vi "DriveModuleControl.vi"(8 "error in":errorcluster, 9 "Actual State":T1={"Speed"=0.0, "Angle"={"VALUE"=0.0, "COS"=1.0, "SIN"=0.0}} {"Angle"."SIN" format="%13.4f"; "Angle"."COS" format="%13.4f"; "Angle"."VALUE" format="%13.4f"}, 10 "Desired State":T1={"Speed"=0.0, "Angle"={"VALUE"=0.0, "COS"=1.0, "SIN"=0.0}} {"Angle"."SIN" format="%13.4f"; "Angle"."COS" format="%13.4f"; "Angle"."VALUE" format="%13.4f"}, 11 "ModualNamePrefix":i32) -> (0 "error out":errorcluster)   [LabVIEW 2023]
uses:
  <vilib>/Rock Robotics/WPI/ThirdParty/JAS_Junk/TrajLib/TypeDef/SWERVE_DRIVE_MODULE_STATE.ctl
  <vilib>/Rock Robotics/WPI/ThirdParty/JAS_Junk/TrajLib/TypeDef/ROTATION2D.ctl
  <vilib>/Rock Robotics/WPI/ThirdParty/JAS_Junk/TrajLib/Rotation2d_Minus.vi
  <vilib>/Rock Robotics/WPI/ThirdParty/JAS_Junk/TrajLib/Rotation2d_GetRadians.vi
  <vilib>/Rock Robotics/WPI/ThirdParty/JAS_Junk/TrajLib/SwerveModuleState_New.vi
  <vilib>/Rock Robotics/WPI/ThirdParty/JAS_Junk/TrajLib/Rotation2d_RotateBy.vi
  <vilib>/Rock Robotics/WPI/ThirdParty/JAS_Junk/TrajLib/Rotation2d_CreateAngle.vi
  <vilib>/Rock Robotics/WPI/ThirdParty/JAS_Junk/TrajLib/SimpleMotorFF_Calculate.vi
  <vilib>/Rock Robotics/WPI/ThirdParty/JAS_Junk/TrajLib/PIDController_AtSetpoint.vi
  <vilib>/Rock Robotics/WPI/ThirdParty/JAS_Junk/TrajLib/PIDController_SetPIDF.vi
  <vilib>/Rock Robotics/WPI/ThirdParty/JAS_Junk/TrajLib/PIDController_SetDerivativeFilter.vi
  <vilib>/Rock Robotics/WPI/ThirdParty/JAS_Junk/TrajLib/PIDController_SetIntegratorRange.vi
  <vilib>/Rock Robotics/WPI/ThirdParty/JAS_Junk/TrajLib/PIDController_SetTolerancePandV.vi
  <vilib>/Rock Robotics/WPI/ThirdParty/JAS_Junk/TrajLib/PIDController_DisableContinousInput.vi
  <vilib>/Rock Robotics/WPI/ThirdParty/JAS_Junk/TrajLib/PIDController_EnableContinousInput.vi
  <vilib>/Rock Robotics/WPI/ThirdParty/JAS_Junk/TrajLib/PIDController_Reset.vi
  <vilib>/Rock Robotics/WPI/ThirdParty/JAS_Junk/TrajLib/PIDController_New.vi
  <vilib>/Rock Robotics/WPI/ThirdParty/JAS_Junk/TrajLib/PIDController_SetOutputLimits.vi
  <vilib>/Rock Robotics/WPI/ThirdParty/JAS_Junk/TrajLib/VI/PIDController_SetIntegratorZone.vi
  <vilib>/Rock Robotics/WPI/ThirdParty/JAS_Junk/TrajLib/SlewRateLimiter_New.vi
  <vilib>/Rock Robotics/WPI/ThirdParty/JAS_Junk/TrajLib/SlewRateLimiter_Reset.vi
  <vilib>/Rock Robotics/WPI/ThirdParty/JAS_Junk/TrajLib/SlewRateLimiter_Calculate.vi
  <vilib>/Rock Robotics/WPI/ThirdParty/JAS_Junk/TrajLib/SlewRateLimiter_SetRate.vi
  <vilib>/Rock Robotics/WPI/ThirdParty/JAS_Junk/TrajLib/Rotation2d_UnaryMinus.vi
  <vilib>/Rock Robotics/WPI/ThirdParty/JAS_Junk/TrajLib/Rotation2d_CreateXY.vi
  <vilib>/Rock Robotics/WPI/ThirdParty/JAS_Junk/TrajLib/PIDController_NewPeriod.vi
  <vilib>/Rock Robotics/WPI/ThirdParty/JAS_Junk/TrajLib/Util_GetTime.vi
  <vilib>/Rock Robotics/WPI/ThirdParty/JAS_Junk/TrajLib/Util_CalcDist.vi
  <vilib>/Rock Robotics/SystemInterfaces/NetworkCommunication/NetComm_UsageReport_report.vi
  <vilib>/Rock Robotics/WPI/ThirdParty/JAS_Junk/TrajLib/VI/Util_GetTime_U32.vi
  DriveGlobal.vi
  <vilib>/Rock Robotics/SystemInterfaces/Utilities/FPGA_UtilitiesRead LocalTime.vi
  <vilib>/Rock Robotics/WPI/ThirdParty/JAS_Junk/TrajLib/VI/Util_GetTime_U64.vi
  <vilib>/Rock Robotics/WPI/ThirdParty/Phoenix6/Phoenix6_Device_RefNumRegistryGet.vi
  <vilib>/Rock Robotics/WPI/MotorControl/WPI_MotorControlRefNum Registry Get.vi
  <vilib>/Rock Robotics/WPI/ThirdParty/JAS_Junk/TrajLib/Globals/Util_LibraryGlobals.vi
  <vilib>/Rock Robotics/WPI/ThirdParty/JAS_Junk/TrajLib/PIDController_AdvCalculate_FF_Sp_Pv.vi
  <vilib>/Rock Robotics/WPI/ThirdParty/JAS_Junk/TrajLib/Trajectory_Library.lvlib
  <vilib>/Rock Robotics/Network Tables/NT Write Number.vi
  <vilib>/Rock Robotics/WPI/ThirdParty/REV Robotics/REVLib/Typedef/Spark MAX Control Type.ctl
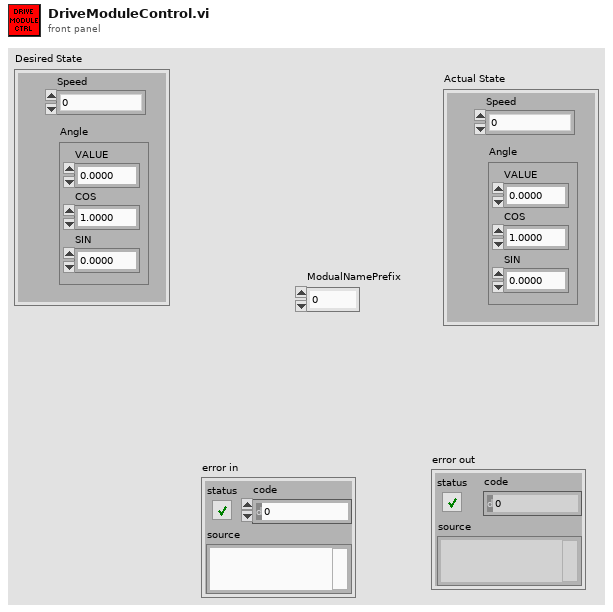
[diagram p1: front panel]
types:
  T1 = typedef "Trajectory_Library.lvlib/SWERVE_DRIVE_MODULE_STATE.ctl" = cluster{"Speed":dbl, "Angle":T2}
  T2 = typedef "Trajectory_Library.lvlib/ROTATION2D.ctl" = cluster{"VALUE":dbl, "COS":dbl, "SIN":dbl}
  T3 = typedef "Spark MAX Control Type.ctl" = enum16{"Percent VBus", "Voltage", "Velocity", "Position", "Smart Motion", "Current", "Smart Velocity", "MAXMotion Position", "MAXMotion Velocity"}
  T4 = typedef "WPI_MotorControlDeviceRef.ctl" = cluster{"DeviceStatus":errorcluster, "Type":T5, "PWM":cluster{"PWM Channel":T6, "DeadBand":T7}, "CAN":cluster{"Device Number":u8, "SetOutput VI Ref":variant, "GetOutput VI Ref":variant, "Enable VI Ref":variant, "Disable VI Ref":variant, "Data":variant}, "Invert":bool, "DIO PWM":cluster{"PWM \"Enable\" Channel":T6, "DIOChannel":T8, "PWM Rate":dbl}}
  T5 = typedef "WPI_MotorControlType.ctl" = enum16{"PWM", "CAN", "DIO PWM"}
  T6 = typedef "FPGA_DIOPWMChannel.ctl" = enum8{"PWM 0", "PWM 1", "PWM 2", "PWM 3", "PWM 4", "PWM 5", "PWM 6", "PWM 7", "PWM 8", "PWM 9", "PWM MXP 0", "PWM MXP 1", "PWM MXP 2", "PWM MXP 3", "PWM MXP 4", "PWM MXP 5", "PWM MXP 6", "PWM MXP 7", "PWM MXP 8", "PWM MXP 9", "Invalid"}
  T7 = typedef "WPI_PWMDeadband.ctl" = cluster{"Name":string, "maxPositivePwm":i32, "minPositivePwm":i32, "centerPwm":i32, "maxNegativePwm":i32, "minNegativePwm":i32, "angularRange":u16}
  T8 = typedef "FPGA_DIOChannel.ctl" = enum8{"DIO 0", "DIO 1", "DIO 2", "DIO 3", "DIO 4", "DIO 5", "DIO 6", "DIO 7", "DIO 8", "DIO 9", "DIO MXP 0", "DIO MXP 1", "DIO MXP 2", "DIO MXP 3", "DIO MXP 4", "DIO MXP 5", "DIO MXP 6", "DIO MXP 7", "DIO MXP 8", "DIO MXP 9", "DIO MXP 10", "DIO MXP 11", "DIO MXP 12", "DIO MXP 13", "DIO MXP 14", "DIO MXP 15", "SPI Port CS1", "SPI Port CS2", "SPI Port CS3", "SPI Port MISO", "SPI Port MOSI", "Invalid"}
  T9 = typedef "Trajectory_Library.lvlib/SIMPLE_MOTOR_FF.ctl" = cluster{"Ks":dbl, "Kv":dbl, "Ka":dbl, "KnInv":dbl}
  T10 = typedef "Trajectory_Library.lvlib/PID_ADV_LIMITS.ctl" = cluster{"MaxInput":dbl, "MinInput":dbl, "Continuous":bool, "MaxOutput":dbl, "MinOutput":dbl}
  T11 = typedef "Trajectory_Library.lvlib/PID_ADV_TUNING.ctl" = cluster{"Kf":dbl, "Kp":dbl, "Ki":dbl, "Kd":dbl, "MaximumIntegral":dbl, "MinimumIntegral":dbl, "Filter Derivative":bool, "IntegralZone":dbl}
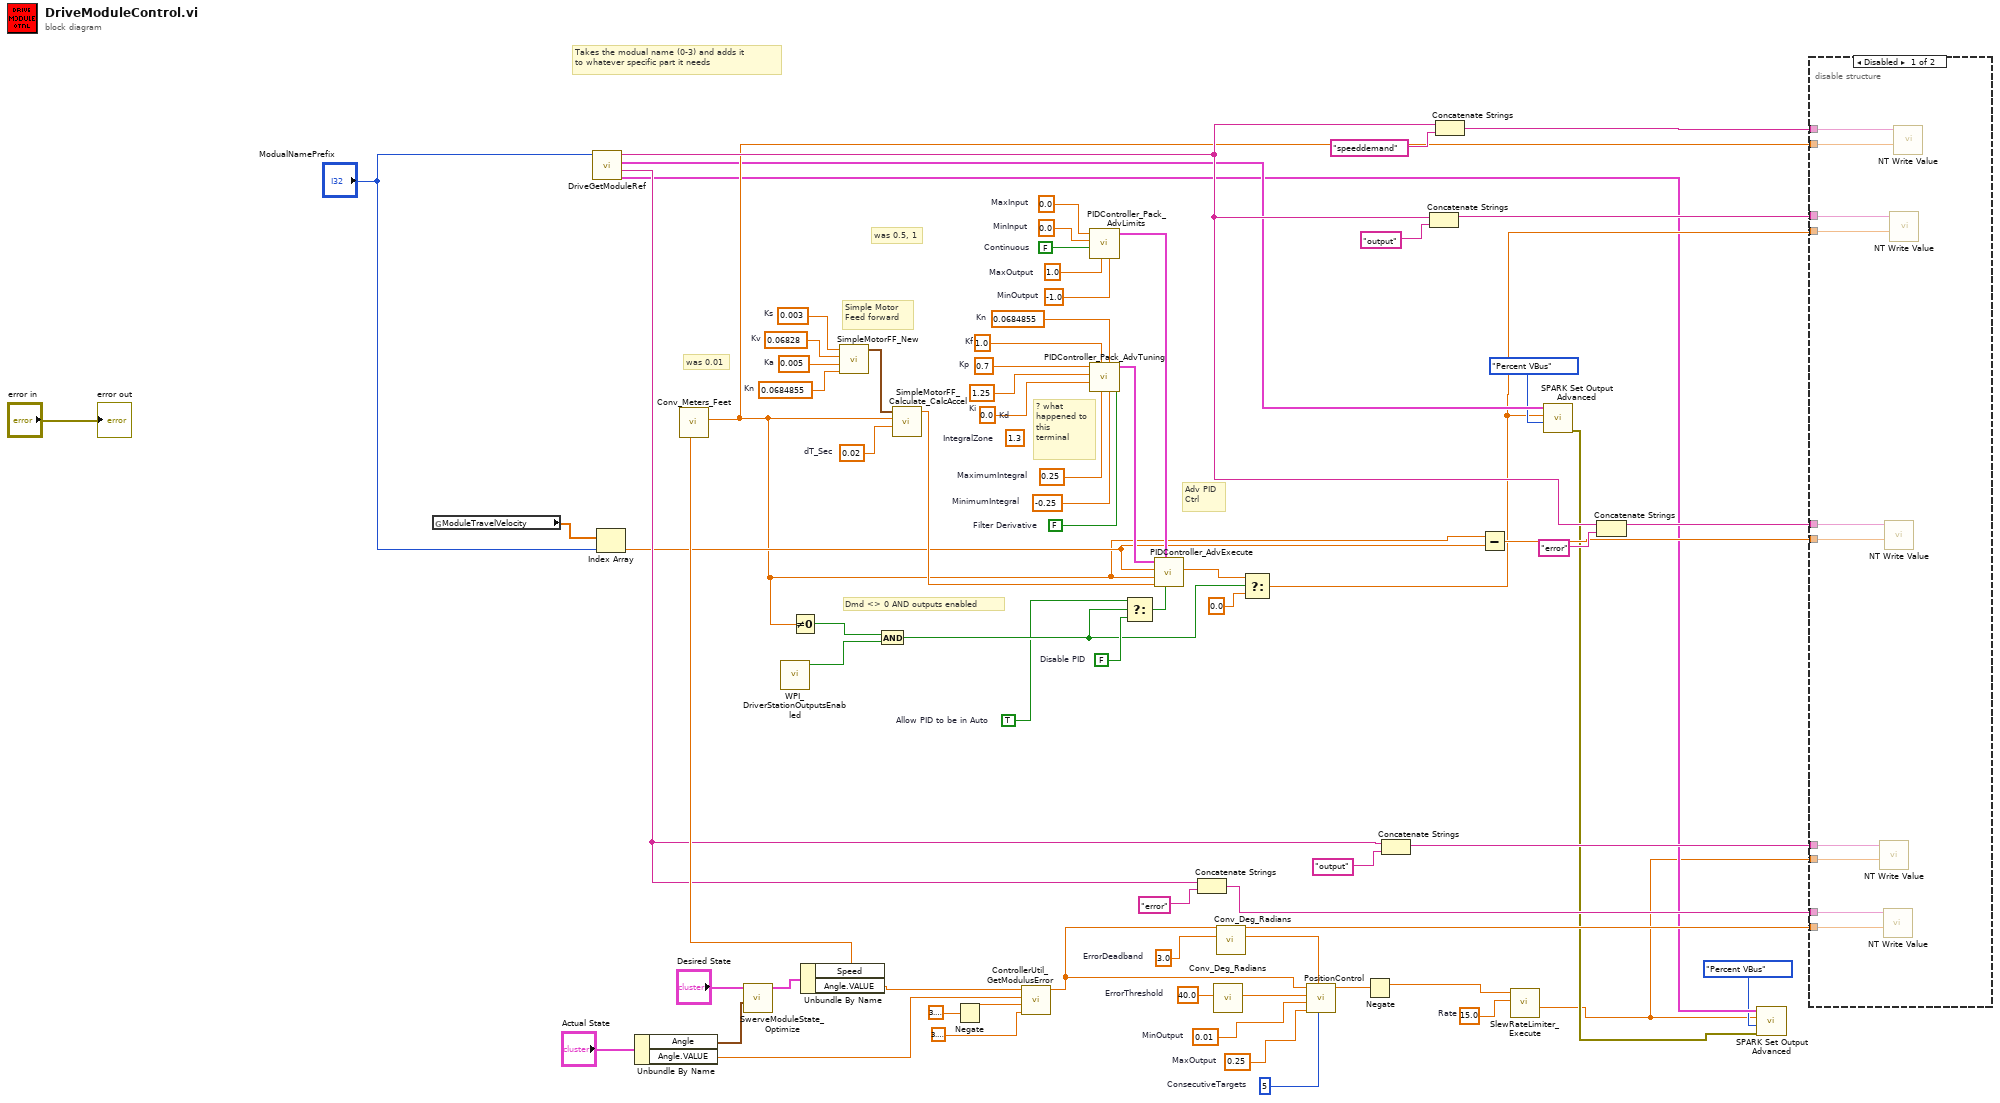
[diagram p0: block diagram]
diagram:
  (unwired) 1.3  # IntegralZone
  w9 = 15.0  # Rate
  w10 = TRUE  # Allow PID to be in Auto
  w12 = FALSE  # Disable PID
  w24 = 0.0684855  # Kn
  w41 = 0.7  # Kp
  w40 = 1.25  # Ki
  w39 = 0.0  # Kd
  w38 = 1.0  # Kf
  w37 = 0.25  # MaximumIntegral
  w36 = -0.25  # MinimumIntegral
  w35 = FALSE  # Filter Derivative
  w33 = 0.0  # MinInput
  w32 = FALSE  # Continuous
  w31 = 1.0  # MaxOutput
  w34 = -1.0  # MinOutput
  w30 = 0.0  # MaxInput
  w48 = 0.0684855  # Kn
  w47 = 0.02  # dT_Sec
  w45 = 0.003  # Ks
  w44 = 0.06828  # Kv
  w43 = 0.005  # Ka
  w58 = 5  # ConsecutiveTargets
  w55 = 0.25  # MaxOutput
  w59 = 0.01  # MinOutput
  w52 = 40.0  # ErrorThreshold
  w54 = 3.0  # ErrorDeadband
  # "was 0.01"
  # "? what happened to this terminal"
  # "was 0.5, 1"
  # "Dmd <> 0 AND outputs enabled"
  # "Adv PID\nCtrl"
  # "Simple Motor\nFeed forward"
  # "Takes the modual name (0-3) and adds it \nto whatever specific part it needs"
  n1 = global read "DriveGlobal.vi" "ModuleTravelVelocity"() -> (w26:dbl[])
  n2 = call "DriveGetModuleRef.vi"("ModualNamePrefix"="ModualNamePrefix") -> ("SpinMot"=w3:T4, "SpinStr"=w42:string, "TravMot"=w7:T4, "TravStr"=w19:string)  [unwired: 5 in, 2 out]
  n3 = Index Array(array=w26, index="ModualNamePrefix") -> (element=w23:dbl)
  n4 = Unbundle By Name("Actual State") -> ("Angle"=w66:T2, "Angle.VALUE"=w62:dbl)
  n5 = call <vilib>:"SwerveModuleState_Optimize.vi"("CurrentAngle"=w66, "Desired State"="Desired State") -> ("out SWERVE_DRIVE_MODULE_STATE"=w64:T1)  [unwired: 9 in]
  n6 = call <vilib>:"WPI_DriverStationOutputsEnabled.vi"() -> ("OutputsEnabled?"=w15:bool)  [unwired: 10 in, 1 out]
  n7 = Unbundle By Name(w64) -> ("Speed"=w49:dbl, "Angle.VALUE"=w63:dbl)
  n8 = call <vilib>:"Conv_Meters_Feet.vi"("Meters"=w49) -> ("Feet"=w18:dbl)  [unwired: 10 in]
  n9 = Not Equal To 0?(x=w18) -> (x != 0?=w14:bool)
  n10 = call <vilib>:"SimpleMotorFF_New.vi"("Kn"=w48, "Ka"=w43, "Kv"=w44, "Ks"=w45) -> ("SIMPLE_MOTOR_FF"=w46:T9)  [unwired: 7 in]
  n11 = And(x=w14, y=w15) -> (x .and. y?=w11:bool)
  n12 = call <vilib>:"SimpleMotorFF_Calculate_CalcAccel.vi"("dT_Sec"=w47, "VelSp"=w18, "SIMPLE_MOTOR_FF"=w46) -> ("FeedForward"=w27:dbl)  [unwired: 8 in]
  n13 = Negate(x=3.141592653589793) -> (-x=w65:dbl)
  n14 = call <vilib>:"ControllerUtil_GetModulusError.vi"("Maximum_Input"=3.141592653589793, "Minimum_Input"=w65, "Measurerment(PV)"=w62, "Reference(SP)"=w63) -> ("Error"=w56:dbl)  [unwired: 7 in]
  n15 = call <vilib>:"PIDController_Pack_AdvLimits.vi"("MinOutput"=w34, "MaxOutput"=w31, "Continuous"=w32, "MinInput"=w33, "MaxInput"=w30) -> ("Adv PID Limits"=w28:T10)  [unwired: 6 in]
  n16 = call <vilib>:"PIDController_Pack_AdvTuning.vi"("Filter Derivative"=w35, "MinimumIntegral"=w36, "Kn"=w24, "MaximumIntegral"=w37, "Kf"=w38, "Kd"=w39, "Ki"=w40, "Kp"=w41) -> ("Adv PID Tuning"=w29:T11)  [unwired: 3 in]
  n17 = Select(t=w10, s=w11, f=w12) -> (s? t:f=w13:bool)
  n18 = call <vilib>:"PIDController_AdvExecute.vi"("Auto"=w13, "Adv PID Limits"=w28, "FF-FeedForward"=w27, "SP-SetPoint"=w18, "PV-Measurement"=w23, "Adv PID Tuning"=w29) -> ("CO-ControlOutput"=w17:dbl)  [unwired: 3 in, 2 out]
  n19 = Concatenate Strings(w42, "error" ("refnum name")) -> (w70:string)
  n20 = call <vilib>:"Conv_Deg_Radians.vi"("Degress"=w52) -> ("Radians"=w51:dbl)  [unwired: 10 in]
  n21 = call <vilib>:"Conv_Deg_Radians.vi"("Degress"=w54) -> ("Radians"=w53:dbl)  [unwired: 10 in]
  n22 = Select(t=w17, s=w11, f=0.0 ("t")) -> (s? t:f=w5:dbl)
  n23 = call "PositionControl.vi"("ConsecutiveTargets"=w58, "ErrorDeadband"=w53, "MaxOutput"=w55, "MinOutput"=w59, "ErrorThreshold"=w51, "Error"=w56) -> ("OutputValue"=w50:dbl)  [unwired: 3 in, 2 out]
  n24 = Negate(x=w50) -> (-x=w8:dbl)
  n25 = Concatenate Strings(w42, "output" ("refnum name")) -> (w57:string)
  n26 = Concatenate Strings(w19, "output" ("refnum name")) -> (w72:string)
  n27 = Concatenate Strings(w19, "speeddemand" ("refnum name")) -> (w74:string)
  n28 = Subtract(x=w18, y=w23) -> (x-y=w20:dbl)
  n29 = call <vilib>:"SlewRateLimiter_Execute.vi"("PositiveRate"=w9, "Input"=w8) -> ("Output"=w1:dbl)  [unwired: 8 in, 1 out]
  n30 = call <vilib>:"SPARK Set Output Advanced.vi"("Control Mode"=Spark_MAX_Control_Type."Percent VBus", "Setpoint"=w5, "MotorControlDevRef"=w7) -> ("error out"=w4:errorcluster)  [unwired: 7 in, 1 out]
  n31 = Concatenate Strings(w19, "error" ("refnum name")) -> (w21:string)
  n32 = call <vilib>:"SPARK Set Output Advanced.vi"("error in (no error)"=w4, "Control Mode"=Spark_MAX_Control_Type."Percent VBus", "Setpoint"=w1, "MotorControlDevRef"=w3) -> ()  [unwired: 6 in, 2 out]
  n33 = disable-structure shown="Disabled" {
    disable-tunnel: w74 -> [w86 _]
    disable-tunnel: w72 -> [w85 _]
    disable-tunnel: w70 -> [w84 _]
    disable-tunnel: w57 -> [w83 _]
    disable-tunnel: w56 -> [w82 _]
    disable-tunnel: w1 -> [w81 _]
    disable-tunnel: w21 -> [w80 _]
    disable-tunnel: w20 -> [w79 _]
    disable-tunnel: w18 -> [w78 _]
    disable-tunnel: w5 -> [w77 _]
    frame Disabled {
      n34 = call-poly <vilib>:"NT Write Value.vi"("value"=w81, "name"=w83) -> ()  [unwired: 9 in, 1 out]
      n35 = call-poly <vilib>:"NT Write Value.vi"("value"=w82, "name"=w84) -> ()  [unwired: 9 in, 1 out]
      n36 = call-poly <vilib>:"NT Write Value.vi"("value"=w79, "name"=w80) -> ()  [unwired: 9 in, 1 out]
      n37 = call-poly <vilib>:"NT Write Value.vi"("value"=w77, "name"=w85) -> ()  [unwired: 9 in, 1 out]
      n38 = call-poly <vilib>:"NT Write Value.vi"("value"=w78, "name"=w86) -> ()  [unwired: 9 in, 1 out]
    }
    frame Enabled {
    }
  }
  "error out" <- "error in"
